vi "Handle Error.vi"(8 "error in (no error)":errorcluster, 11 "CCD Configuration in":refnum<class "CCD Configuration.lvclass">) -> (0 "error out":errorcluster, 2 "stop actor?":bool=TRUE, 3 "CCD Configuration out":refnum<class "CCD Configuration.lvclass">)   [LabVIEW 2016, in "Hardware.lvlib" / "CCD.lvlib" / "CCD Configuration.lvclass"]
doc: "(<B>Filename</B>: Actor Framework.lvlib:Actor.lvclass:Handle Error.vi)\n\nDefines how the actor handles an error that occurred while processing a message. By default, this method does nothing except stop the actor."
uses:
  <userlib>/Common Components/Hardware/CCD/CCD Configuration.lvclass
  <userlib>/Configuration Dialog Actor/Configuration.lvclass
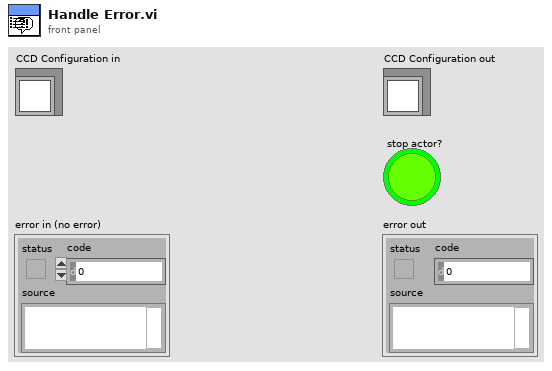
[diagram p1: front panel]
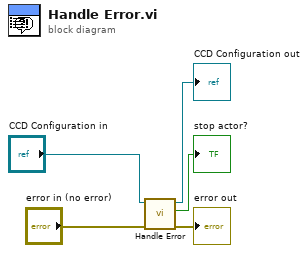
[diagram p0: block diagram]
diagram:
  n1 = call-parent "Handle Error.vi"("error in (no error)"="error in (no error)", "Configuration in"="CCD Configuration in") -> ("error out"=→"error out":errorcluster, "stop actor?"=→"stop actor?":bool, "Configuration out"=→"CCD Configuration out":refnum<class "CCD Configuration.lvclass">)  [unwired: 7 in]
